vi "FarFiledDefineOffset.vi"(6 "正序？":bool, 7 "状态":enum16{"计算总分辨率", "计算偏移量"}(ring), 8 "当前Y位置":i32, 9 "当前X位置":i32, 10 "Y Pos Num":i32, 11 "X Pos Num":i32) -> (0 "offset":i32[](array[numeric]), 1 "Y Resolution":i32, 2 "X Resolution":i32, 3 "单个分辨率":i32)   [LabVIEW 2018]
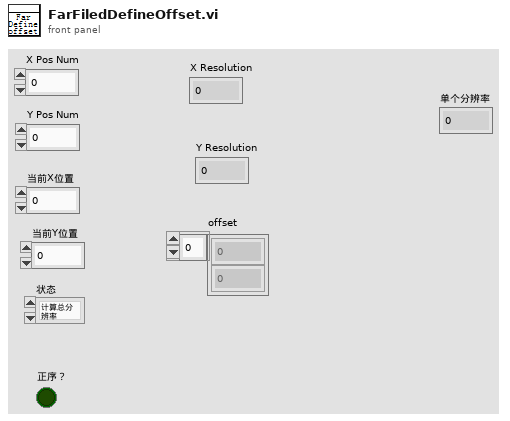
[diagram p1: front panel]
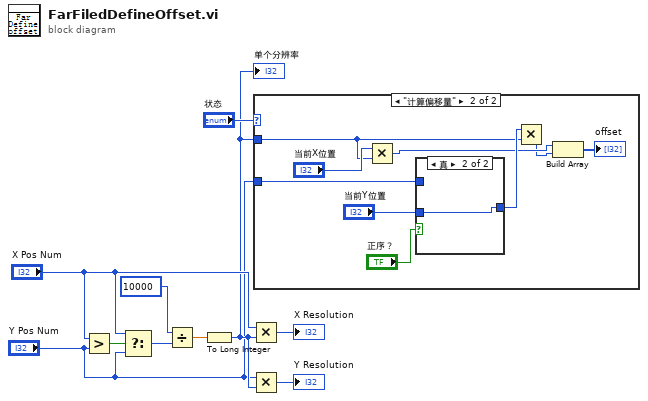
[diagram p0: block diagram]
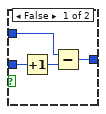
[diagram p3: hidden frame]
diagram:
  n1 = Greater?(x="X Pos Num", y="Y Pos Num") -> (0:w4:bool)
  n2 = Select(t="X Pos Num", s=w4, f="Y Pos Num") -> (s? t:f=w5:i32)
  n3 = Divide(x=10000, y=w5) -> (x/y=w6:dbl)
  n4 = To Long Integer(number=w6) -> (32bit integer=w2:i32)
  "单个分辨率" <- w2
  n5 = Multiply(x="X Pos Num", y=w2) -> (x*y=→"X Resolution":i32)
  n6 = Multiply(x="Y Pos Num", y=w2) -> (x*y=→"Y Resolution":i32)
  n7 = case shown="\"计算偏移量\"" "状态" {
    tunnel: w2 -> [_ w14]
    tunnel: "Y Pos Num" -> [_ w15]
    frame "计算总分辨率", Default {
    }
    frame "计算偏移量" {
      n8 = Multiply(x="当前X位置", y=w14) -> (x*y=w12:i32)
      n9 = case shown="真" "正序？" {
        tunnel: "当前Y位置" -> [w23 w24]
        tunnel: [w20 w24] -> w16
        tunnel: w15 -> [w22 _]
        frame False {
          n10 = Increment(x=w23) -> (x+1=w21:i32)
          n11 = Subtract(x=w22, y=w21) -> (x-y=w20:i32)
        }
        frame True {
        }
      }
      n12 = Multiply(x=w16, y=w14) -> (x*y=w11:i32)
      n13 = Build Array(w12, w11) -> (→"offset":i32[])
    }
  }
